vi "Read Read Only.vi"(8 "error in (no error)":errorcluster, 11 "Const_Variant in":refnum<class "Const_Variant_1D.lvclass">) -> (0 "error out":errorcluster, 2 "Read Only":bool, 3 "Const_Variant out":refnum<class "Const_Variant_1D.lvclass">)   [LabVIEW 2021, in "Const_Variant_1D.lvclass"]
uses:
  Const_Variant_1D.lvclass
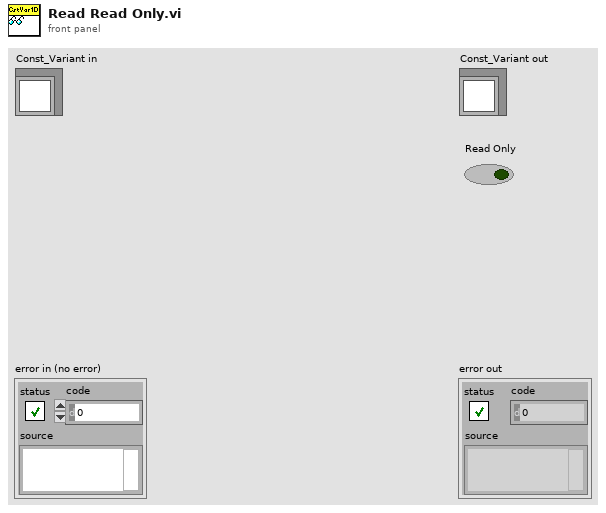
[diagram p1: front panel]
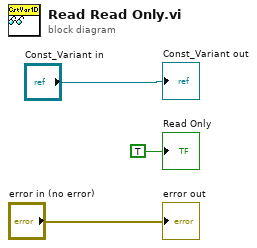
[diagram p0: block diagram]
diagram:
  "error out" <- "error in (no error)"
  "Const_Variant out" <- "Const_Variant in"
  "Read Only" <- TRUE ("Read Only")
